vi "TEMPLATE Output.vi"(8 "Error in":errorcluster, 9 "Teller":T2 {"Absolute Time" format="%<%x %.3X>T"}, 10 "Output in":T1, 11 "TEMPLATE jettl Msg in":refnum<class "TEMPLATE jettl Msg.lvclass">) -> (0 "Error out":errorcluster, 2 "Output out":T1, 3 "TEMPLATE jettl Msg out":refnum<class "TEMPLATE jettl Msg.lvclass">)   [LabVIEW 2020, in "_Template.lvlib" / "Templates.lvlib" / "TEMPLATE jettl Msg.lvlib" / "TEMPLATE jettl Msg.lvclass"]
uses:
  TEMPLATE jettl Msg.lvclass
  jettl/jettl/Unified Actor Relation.ctl
  jettl/jettl/jettl.lvlib
  jettl/jettl/Teller.ctl
  Output.ctl
  TEMPLATE jettl Msg.lvlib
panel:
  # "This front panel should not be manipulated."
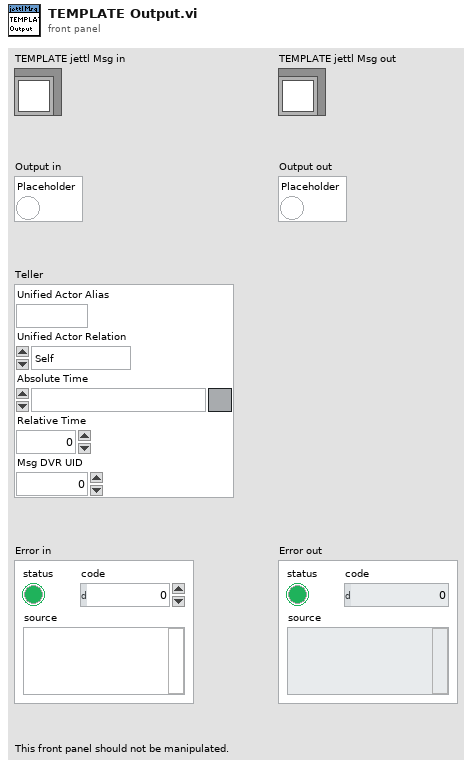
[diagram p1: front panel]
types:
  T1 = typedef "_Template.lvlib/Templates.lvlib/TEMPLATE jettl Msg.lvlib/Output.ctl" = cluster{"Placeholder":bool}
  T2 = typedef "jettl.lvlib/Teller.ctl" = cluster{"Unified Actor Alias":string, "Unified Actor Relation":T3, "Absolute Time":timestamp, "Relative Time":dbl, "Msg DVR UID":i32}
  T3 = typedef "jettl.lvlib/Unified Actor Relation.ctl" = enum16{"Self", "Parent", "Child"}
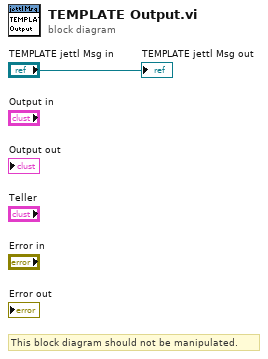
[diagram p0: block diagram]
diagram:
  # "This block diagram should not be manipulated."
  "TEMPLATE jettl Msg out" <- "TEMPLATE jettl Msg in"
